vi "ParseArgumentsCore.vi"(8 "error in (no error)":errorcluster, 9 "Value":string, 10 "Option":string, 11 "ExecuteAllBuildSpecsWithVersion in":refnum<class "ExecuteAllBuildSpecsWithVersion.lvclass">) -> (0 "error out":errorcluster, 3 "ExecuteAllBuildSpecsWithVersion out":refnum<class "ExecuteAllBuildSpecsWithVersion.lvclass">)   [LabVIEW 2015, in "ExecuteAllBuildSpecsWithVersion.lvclass"]
doc: "VI to be overridden by child classes to parse operation-specific arguments."
uses:
  ExecuteAllBuildSpecsWithVersion.lvclass
  <nishared>/LabVIEW CLI/Operations/Utilities/OperationErrorType.ctl
  ExecuteAllBuildSpecsWithVersion.lvclass/ExecuteAllBuildSpecsWithVersion.ctl
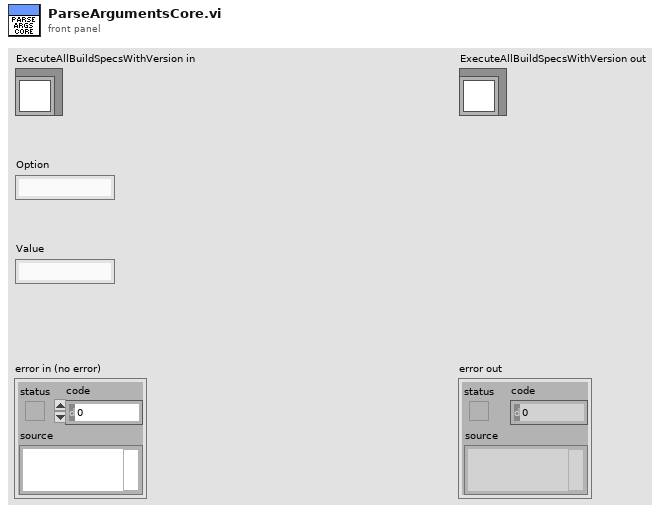
[diagram p1: front panel]
types:
  T1 = typedef "OperationErrorType.ctl" = enum16{"RequiredArgumentMissing", "UnknownArguments", "LoggerSetMultipleTimes", "OperationBrokenError"}
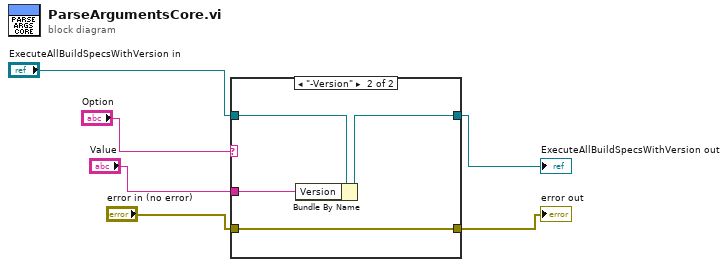
[diagram p0: block diagram]
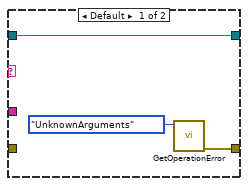
[diagram p2: hidden frame]
diagram:
  n1 = case shown="\"-Version\"" "Option" {
    tunnel: "error in (no error)" -> [_ w13]
    tunnel: [w7 w13] -> w4
    tunnel: "Value" -> [_ w12]
    tunnel: "ExecuteAllBuildSpecsWithVersion in" -> [w9 w11]
    tunnel: [w9 w10] -> w5
    frame Default {
      n2 = call <nishared>:"GetOperationError.vi"("Operation Error Type"=OperationErrorType."UnknownArguments") -> ("error out"=w7:errorcluster)  [unwired: 10 in]
    }
    frame "-Version" {
      n3 = Bundle By Name(cluster=w11, "Version"=w12) -> (w10:refnum<class "ExecuteAllBuildSpecsWithVersion.lvclass">)
    }
  }
  "error out" <- w4
  "ExecuteAllBuildSpecsWithVersion out" <- w5
